vi "Initialize.vi"(6 "optional":variant, 8 "error in":errorcluster, 11 "U32 in":refnum<class "U32.lvclass">) -> (0 "error out":errorcluster, 3 "Node*":refnum<data-value>)   [LabVIEW 2014, in "U32.lvclass"]
doc: "Initializes a node. Makes a data value reference of the node, sets the selfNode, and output the data value reference."
uses:
  U32.lvclass
  xCE/xceNode/xceNode.lvclass
  xCE/xceDataNode/xceDataNode.lvclass
  FPGADMAChannelData/PWM_Specific Data.ctl
  Channel/Channel.lvclass
  FPGADMAChannelData/FPGADMAChannelData.lvclass
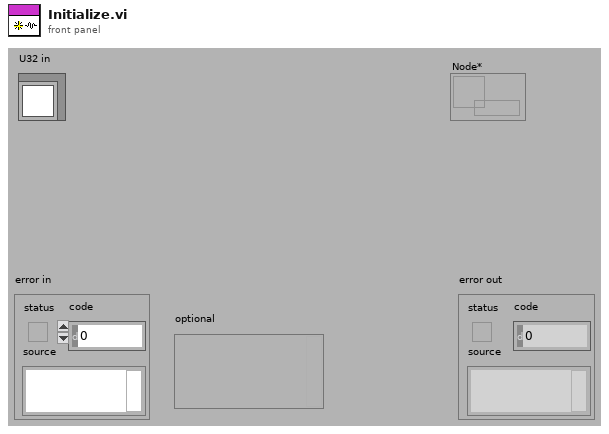
[diagram p1: front panel]
types:
  T1 = typedef "FPGADMAChannelData.lvclass/PWM_Specific Data.ctl" = cluster{"# of parameters":i32, "CnfgEditorDir":path}
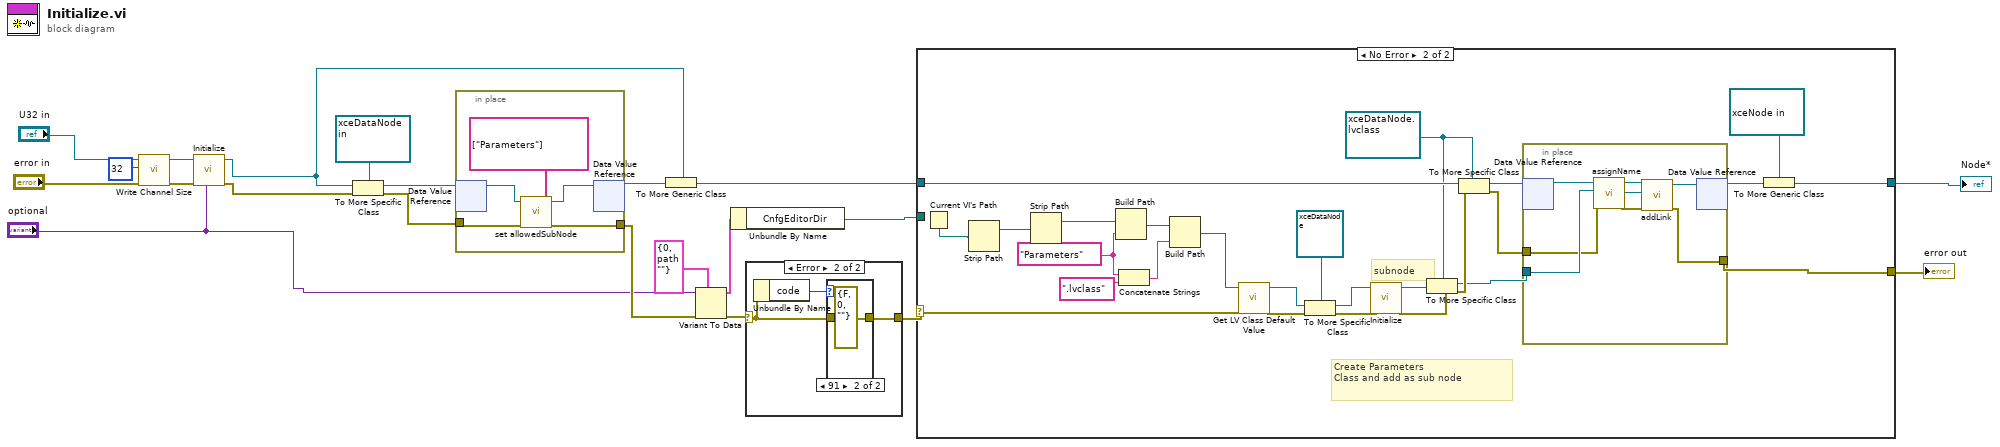
[diagram p0: block diagram]
diagram:
  n1 = call "Write Channel Size.vi"("error in (no error)"="error in", "Channel Size"=32, "Channel in"="U32 in") -> ("error out"=w20:errorcluster, "Channel out"=w19:refnum<class "U32.lvclass">)  [unwired: 7 in]
  n2 = call-parent "Initialize.vi"("optional"="optional", "error in"=w20, "Channel in"=w19) -> ("error out"=w5:errorcluster, "Node*"=w4:refnum<data-value>)  [unwired: 7 in]
  n3 = To More Specific Class(target class=refnum<data-value> refnum ("data value reference"), reference=w4, error in=w5) -> (specific class reference=w6:refnum<data-value>, error out=w7:errorcluster)
  n4 = in-place {
    in-place-border: w7 -> [w23]
    in-place-border: [w22] -> w11
    n5 = in-place-dvr #1(w6) -> (w25:refnum<class "xceDataNode.lvclass">)  [unwired: 1 out]
    n6 = call "set allowedSubNode.vi"("error in (no error)"=w23, "Allowed subNode[]"=string[] ["Parameters"], "xceDataNode in"=w25) -> ("error out"=w22:errorcluster, "xceDataNode out"=w24:refnum<class "xceDataNode.lvclass">)  [unwired: 7 in]
    n7 = in-place-dvr #1(w24) -> (w9:refnum<data-value>)  [unwired: 1 out]
  }
  n8 = To More Generic Class(target class=w4, reference=w9) -> (generic class reference=w13:refnum<data-value>)
  n9 = Variant To Data(error in=w11, type=T1 {"# of parameters"=0, "CnfgEditorDir"=path ""} ("Cluster"), Variant="optional") -> (data=w10:T1, error out=w15:errorcluster)
  n10 = Unbundle By Name(w10) -> ("CnfgEditorDir"=w12:path)
  n11 = case shown="Error" w15 {
    selector: w15 -> [w27 w29]
    tunnel: [w27 w28] -> w16
    frame No Error {
    }
    frame Error {
      n12 = Unbundle By Name(w29) -> ("code"=w30:i32)
      n13 = case shown="91" w30 {
        tunnel: w29 -> [w31 _]
        tunnel: [w31 errorcluster {"status"=FALSE, "code"=0, "source"=""} ("error IO")] -> w28
        frame 0, Default {
        }
        frame 91 {
        }
      }
    }
  }
  n14 = case shown="No Error" w16 {
    selector: w16 -> [w33 w43]
    tunnel: [w34 w46] -> w1
    tunnel: [w33 w44] -> w2
    tunnel: w12 -> [_ _]
    tunnel: w13 -> [w34 w42]
    frame Error {
    }
    frame No Error {
      w41 = refnum<data-value> refnum ("data value reference")
      w57 = "Parameters" ("name or relative path")
      # "subnode"
      # "Create Parameters\nClass and add as sub node"
      n15 = Current VI's Path() -> (path=w37:path)
      n16 = Strip Path(path=w37) -> (stripped path=w36:path)  [unwired: 1 out]
      n17 = Strip Path(path=w36) -> (stripped path=w35:path)  [unwired: 1 out]
      n18 = Build Path(base path=w35, name or relative path=w57) -> (appended path=w59:path)
      n19 = Concatenate Strings(w57, ".lvclass" ("string")) -> (w60:string)
      n20 = Build Path(base path=w59, name or relative path=w60) -> (appended path=w53:path)
      n21 = call <vilib>:"Get LV Class Default Value.vi"("error in (no error)"=w43, "class path"=w53) -> ("error out"=w56:errorcluster, "object"=w54:refnum<class>)  [unwired: 8 in]
      n22 = To More Specific Class(target class=refnum<class "xceDataNode.lvclass"> refnum ("xceDataNode.lvclass"), reference=w54, error in=w56) -> (specific class reference=w51:refnum<class "xceDataNode.lvclass">, error out=w52:errorcluster)
      n23 = call-dynamic "Initialize.vi"("error in"=w52, "xceDataNode in"=w51) -> ("error out"=w49:errorcluster, "Node*"=w50:refnum<data-value>)  [unwired: 8 in]
      n24 = To More Specific Class(target class=w41, reference=w50, error in=w49) -> (specific class reference=w47:refnum<data-value>, error out=w48:errorcluster)
      n25 = To More Specific Class(target class=w41, reference=w42, error in=w48) -> (specific class reference=w39:refnum<data-value>, error out=w40:errorcluster)
      n26 = in-place {
        in-place-border: w47 -> [w68]
        in-place-border: w40 -> [w67]
        in-place-border: [w63] -> w44
        n27 = in-place-dvr #2(w39) -> (w62:refnum<class "xceDataNode.lvclass">)  [unwired: 1 out]
        n28 = call "assignName.vi"("error in (no error)"=w67, "subNode in"=w68, "superNode in"=w62) -> ("error out"=w64:errorcluster, "subNode out"=w65:refnum<data-value>, "superNode out"=w66:refnum<class "xceDataNode.lvclass">)  [unwired: 6 in]
        n29 = call "addLink.vi"("error in (no error)"=w64, "subNode in"=w65, "superNode in"=w66) -> ("error out"=w63:errorcluster, "superNode out"=w61:refnum<class "xceDataNode.lvclass">)  [unwired: 6 in, 1 out]
        n30 = in-place-dvr #2(w61) -> (w38:refnum<data-value>)  [unwired: 1 out]
      }
      n31 = To More Generic Class(target class=refnum<data-value> refnum ("Node*"), reference=w38) -> (generic class reference=w46:refnum<data-value>)
    }
  }
  "error out" <- w2
  "Node*" <- w1
